vi "createPlatformData_autoRaiseANDLower.vi"(1 "Plaforms to raise":i32[](array[numeric]), 2 "Plaforms to lower":i32[](array[numeric])) -> (8 "platformData":bool[](array[boolean]))   [LabVIEW 2017]
uses:
  <vilib>/imath/engines/lvmath2/RunTimeEngine/BuiltInFunctions/logical/NIMS_logical(A).vi
  <instcachedir>/0/NIMS_logical(A)_4BC617C6B9DD45D5BCECC39AA35EA8BB.lvgen/NIMS_logical(A)_4BC617C6B9DD45D5BCECC39AA35EA8BB_001.vi
  <vilib>/imath/engines/lvmath2/RunTimeEngine/VariableToken/Support/NIMS_Vector Boolean Index to I32 Index.vi
  <vilib>/imath/engines/lvmath2/RunTimeEngine/IndexReplace/NIMS V(V)=M.vi
  <instcachedir>/0/NIMS V(V)=M_0ADE186F28374EB287D72E31354E4201.lvgen/NIMS V(V)=M_0ADE186F28374EB287D72E31354E4201_000.vi
  <vilib>/imathl/engines/lvmath/Functions/Error Handling/Create Error.vi
  <vilib>/imath/engines/lvmath2/RunTimeEngine/BuiltInFunctions/is_empty/NIMS_is_empty(GV).vi
  <instcachedir>/0/NIMS_is_empty(GV)_FC7E7C3D9544432CB6AA2416ADCF6D56.lvgen/NIMS_is_empty(GV)_FC7E7C3D9544432CB6AA2416ADCF6D56_001.vi
  <vilib>/imath/engines/lvmath2/RunTimeEngine/IndexReplace/NIMS V(V)=S.vi
  <instcachedir>/0/NIMS V(V)=S_01936889079944FABA298608ED103678.lvgen/NIMS V(V)=S_01936889079944FABA298608ED103678_001.vi
  <vilib>/imath/engines/lvmath2/RunTimeEngine/MatrixToken/NIMS_MatrixToken_RV_RV.vi
  <instcachedir>/0/NIMS_MatrixToken_RV_RV_8B087EE0EE16477EBE1C341EABB504F3.lvgen/NIMS_MatrixToken_RV_RV_8B087EE0EE16477EBE1C341EABB504F3_002.vi
  <vilib>/imath/engines/lvmath2/RunTimeEngine/IndexRead/NIMS M($).vi
  <instcachedir>/0/NIMS M($)_82D1177398184AFB96A6AFB63C3C3F57.lvgen/NIMS M($)_82D1177398184AFB96A6AFB63C3C3F57_005.vi
  <vilib>/imath/engines/lvmath2/RunTimeEngine/BuiltInFunctions/length/NIMS_length(GV).vi
  <instcachedir>/0/NIMS_length(GV)_08A3D13377FD4E4B96F5795FBF3698FA.lvgen/NIMS_length(GV)_08A3D13377FD4E4B96F5795FBF3698FA_002.vi
  <vilib>/imath/engines/lvmath2/RunTimeEngine/CommandStatement/MC_CommandStatement_break.vi
  <vilib>/imath/engines/lvmath2/RunTimeEngine/IndexRead/NIMS V(S).vi
  <instcachedir>/0/NIMS V(S)_0488751826AF41519A22953C041130DC.lvgen/NIMS V(S)_0488751826AF41519A22953C041130DC_002.vi
  <vilib>/imath/engines/lvmath2/RunTimeEngine/IndexRead/NIMS V(R2).vi
  <instcachedir>/0/NIMS V(R2)_C76619605A0E4E9F8B2FA9389712AC47.lvgen/NIMS V(R2)_C76619605A0E4E9F8B2FA9389712AC47_003.vi
  <vilib>/imath/engines/lvmath2/RunTimeEngine/ErrorHandling/NIMS_Create Error From Enums.vi
  <vilib>/imath/engines/lvmath2/RunTimeEngine/CommandStatement/NIMS_CommandStatement_MaskErr.vi
  <vilib>/imath/engines/lvmath2/RunTimeEngine/NodeEndStatement/NIMS_NodeEndStatement_Output.vi
  <instcachedir>/0/NIMS_NodeEndStatement_Output_53EC0D466D134D7ABD903AC30B43404B.lvgen/NIMS_NodeEndStatement_Output_53EC0D466D134D7ABD903AC30B43404B_011.vi
  <vilib>/imath/engines/lvmath2/RunTimeEngine/ErrorHandling/NIMS_Finalize Error.vi
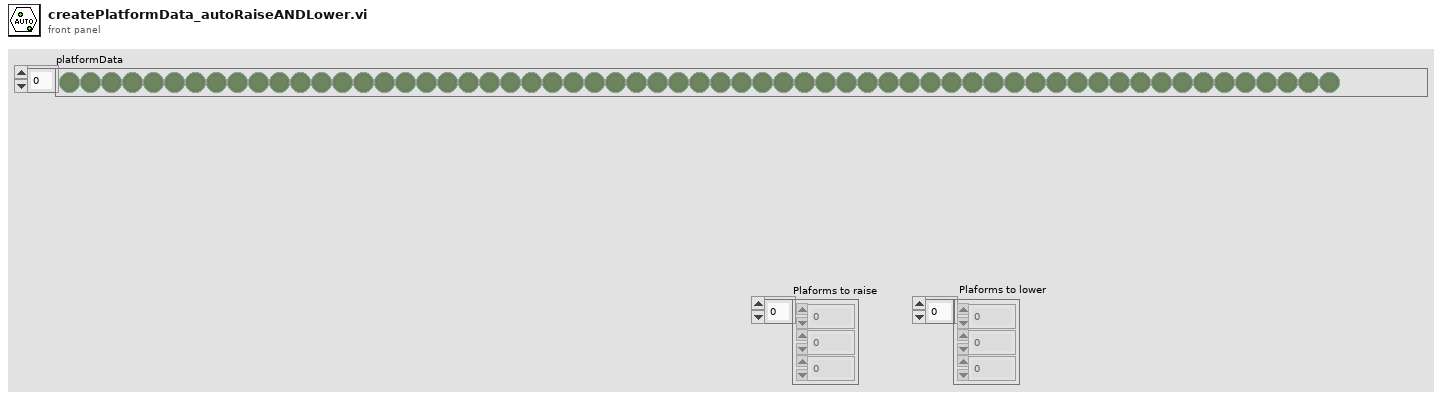
[diagram p1: front panel]
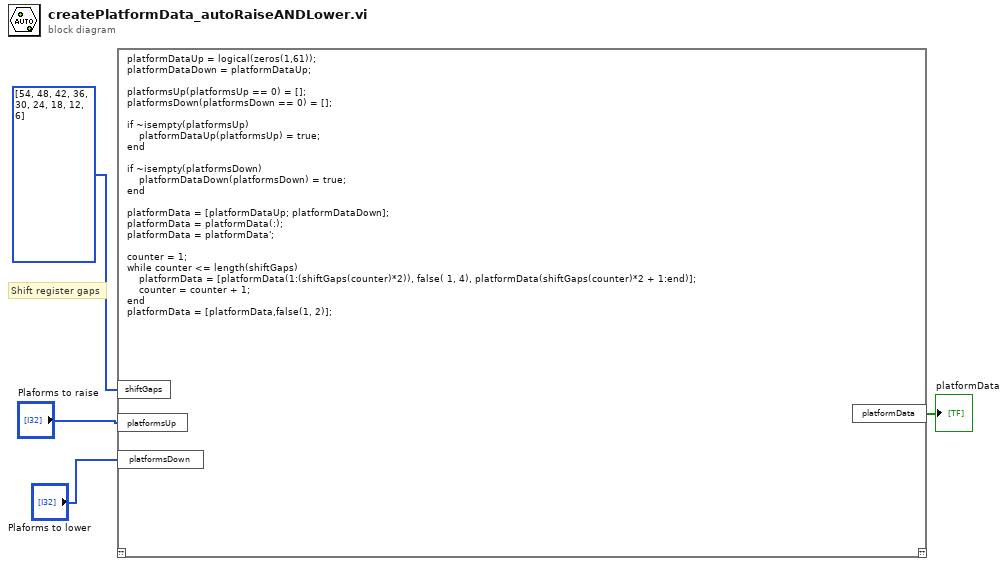
[diagram p0: block diagram]
diagram:
  # "Shift register gaps"
  n1 = mathscript code="platformDataUp = logical(zeros(1,61));\nplatformDataDown = platformDataUp;\n\nplatformsUp(platformsUp == 0) = [];\nplatformsDown(platformsDown == 0) = [];\n\nif ~isempty(platformsUp)\n    platformDataUp(platformsUp) = true;\nend\n\nif ~isempty(platformsDown)\n    platformDataDown(platformsDown) = true;\nend\n\nplatformData = [platformDataUp; platformDataDown];\nplatformData = platformData(:);\nplatformData = platformData';\n\ncounter = 1;\nwhile counter <= length(shiftGaps)\n    platformData = [platformData(1:(shiftGaps(counter)*2)), false( 1, 4), platformData(shiftGaps(counter)*2 + 1:end)];\n    counter = counter + 1;\nend\nplatformData = [platformData,false(1, 2)];"("shiftGaps"=i32[] [54, 48, 42, 36, 30, 24, 18, 12, 6] ("Plaforms to raise 2"), "platformsUp"="Plaforms to raise", "platformsDown"="Plaforms to lower") -> ("platformData"=→"platformData":bool[])  [unwired: 1 in, 1 out]
